vi "score.vi"() -> ()   [LabVIEW 2018]
panel:
  out "output array":bool[](array[boolean])
  out "Boolean 14":bool
  out "Boolean 13":bool
  out "Boolean 12":bool
  out "Boolean 11":bool
  out "Boolean 10":bool
  out "Boolean 9":bool
  out "Boolean 8":bool
  out "Boolean 7":bool
  out "Boolean 6":bool
  out "Boolean 5":bool
  out "Boolean 4":bool
  out "Boolean 3":bool
  out "Boolean 2":bool
  out "Boolean":bool
  out "Array":bool[][](array[boolean])=[[FALSE, FALSE, TRUE, FALSE, FALSE, FALSE, TRUE, FALSE, FALSE, FALSE], [TRUE, TRUE, FALSE, TRUE, FALSE, TRUE, TRUE, FALSE, FALSE, FALSE], [FALSE, TRUE, TRUE, TRUE, FALSE, TRUE, TRUE, FALSE, FALSE, FALSE], [FALSE, FALSE, TRUE, TRUE, TRUE, FALSE, TRUE, FALSE, FALSE, FALSE], [FALSE, TRUE, TRUE, TRUE, TRUE, TRUE, FALSE, FALSE, FALSE, FALSE], [TRUE, TRUE, TRUE, TRUE, TRUE, TRUE, FALSE, FALSE, FALSE, FALSE], [FALSE, FALSE, TRUE, FALSE, FALSE, TRUE, TRUE, TRUE, TRUE, TRUE], [TRUE, TRUE, TRUE, TRUE, TRUE, TRUE, TRUE, TRUE, TRUE, TRUE], [FALSE, TRUE, TRUE, TRUE, TRUE, TRUE, TRUE, TRUE, TRUE, TRUE]]
  in  "Numeric":dbl
  in  "stop":bool
  in  "time":dbl=60.0
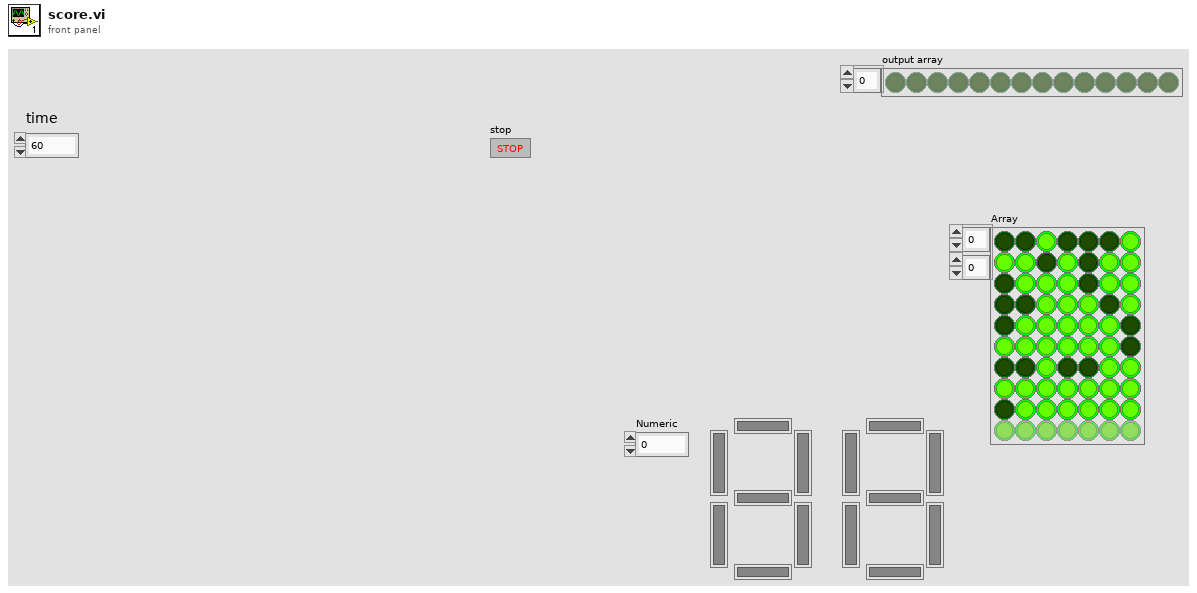
[diagram p1: front panel]
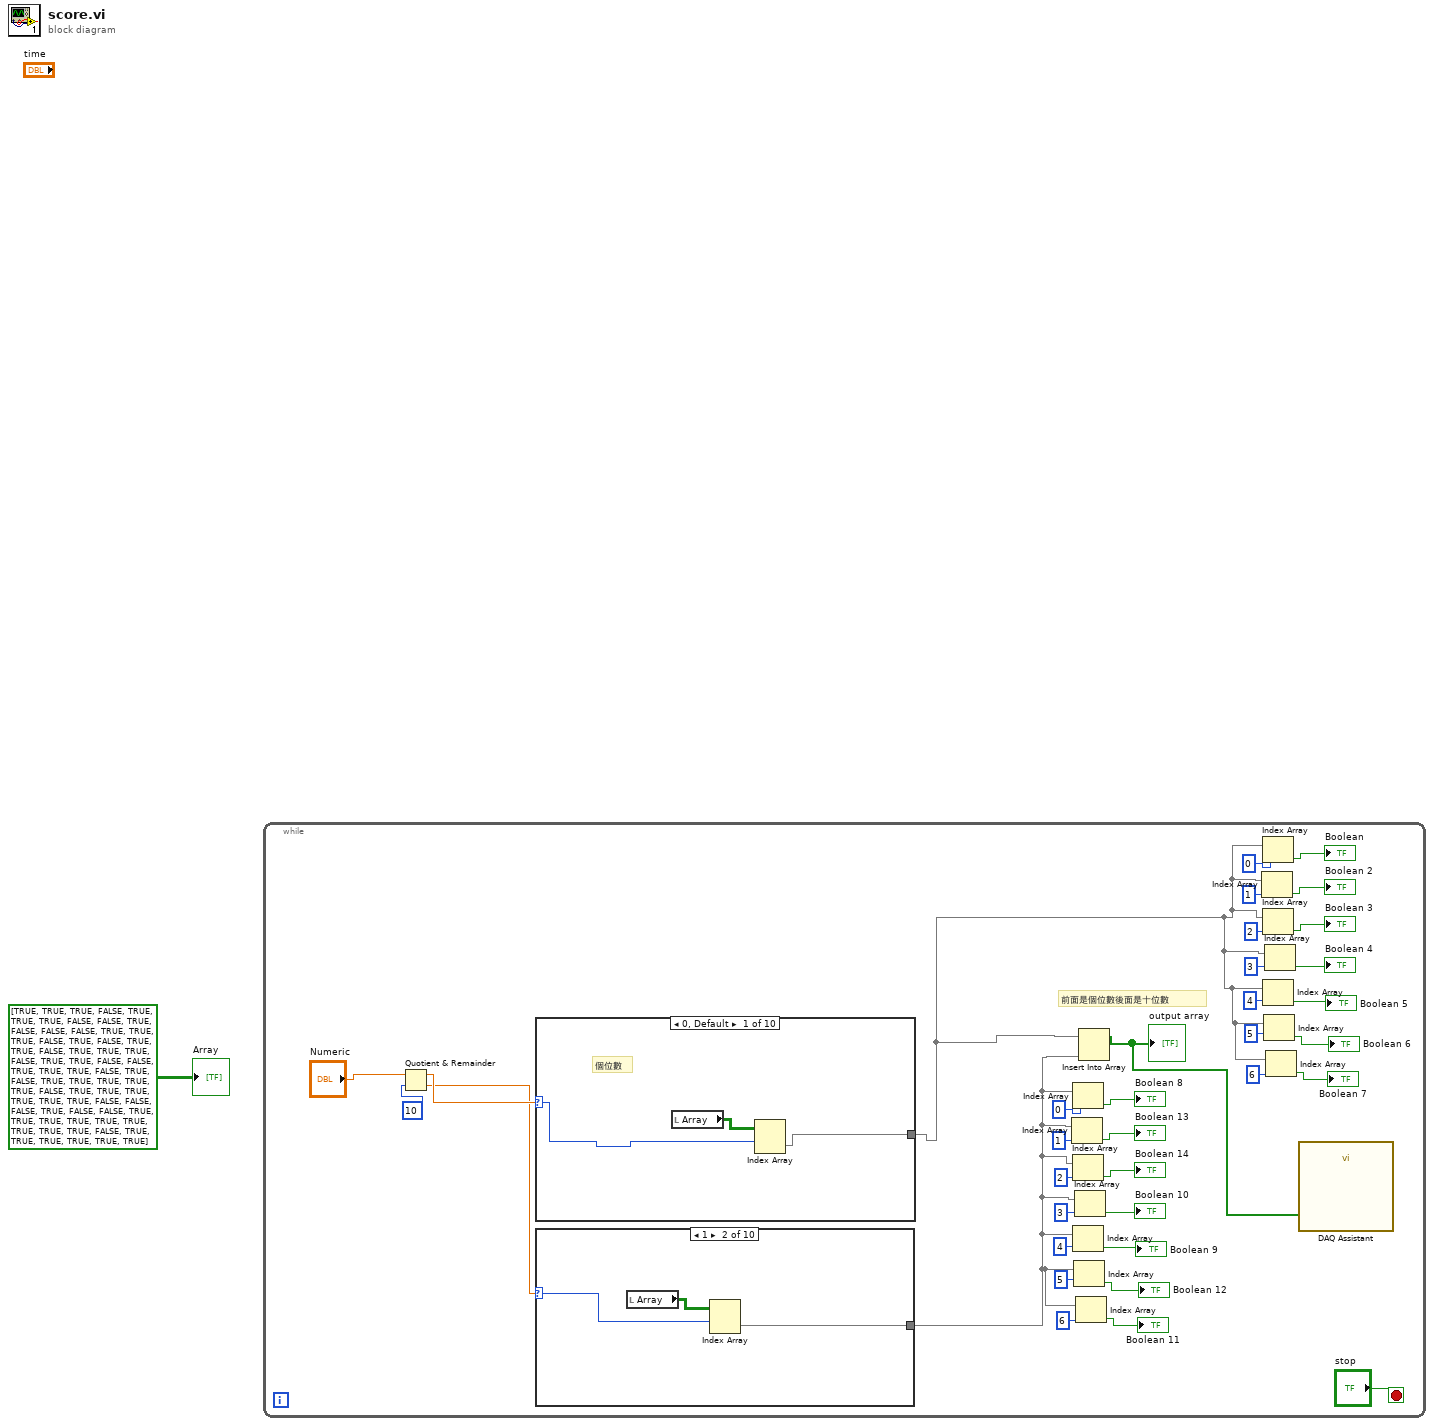
[diagram p0: block diagram]
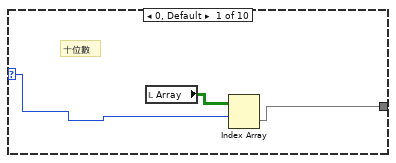
[diagram p2: hidden frame]
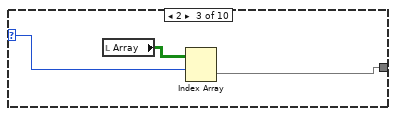
[diagram p3: hidden frame]
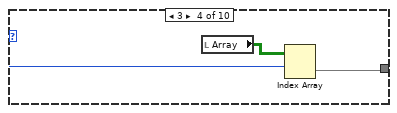
[diagram p4: hidden frame]
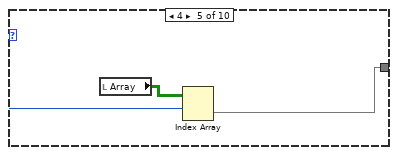
[diagram p5: hidden frame]
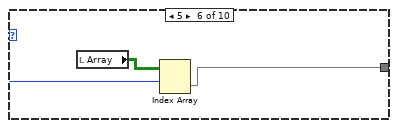
[diagram p6: hidden frame]
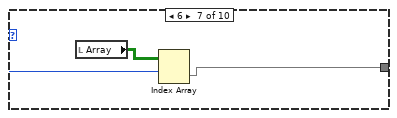
[diagram p7: hidden frame]
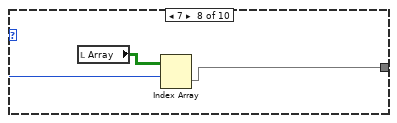
[diagram p8: hidden frame]
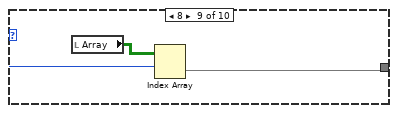
[diagram p9: hidden frame]
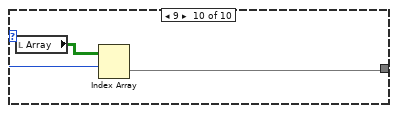
[diagram p10: hidden frame]
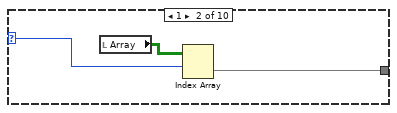
[diagram p11: hidden frame]
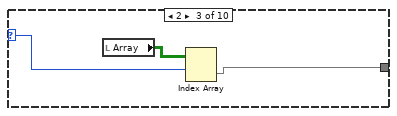
[diagram p12: hidden frame]
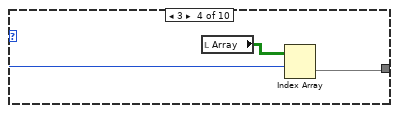
[diagram p13: hidden frame]
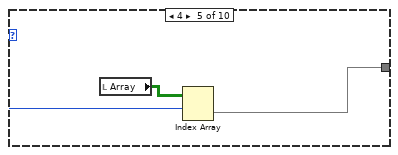
[diagram p14: hidden frame]
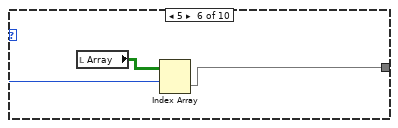
[diagram p15: hidden frame]
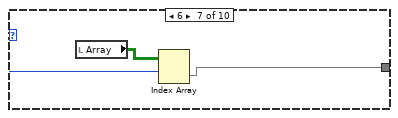
[diagram p16: hidden frame]
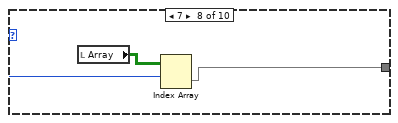
[diagram p17: hidden frame]
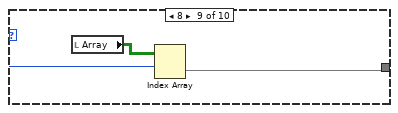
[diagram p18: hidden frame]
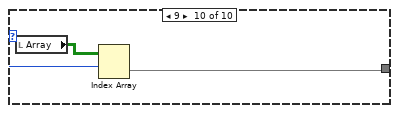
[diagram p19: hidden frame]
diagram:
  n1 = while {
    stop <- "stop" stop-if-true
    # "前面是個位數後面是十位數"
    n2 = Quotient & Remainder(x="Numeric", y=10) -> (x-y*floor(x/y)=w4:dbl, floor(x/y)=w3:dbl)
    n3 = case shown="0, Default" w4 {
      selector: w4 -> [w68 w72 w75 w78 w81 w84 w87 w90 w93 w96]
      tunnel: [w69 w71 w74 w77 w80 w83 w86 w89 w92 w95] -> w6
      frame 0, Default {
        # "個位數"
        n4 = local read "Array"() -> (w70:bool[][])
        n5 = Index Array(array=w70, index (row)=w68) -> (element=w69:bool[])  [unwired: 1 in]
      }
      frame 1 {
        n6 = local read "Array"() -> (w73:bool[][])
        n7 = Index Array(array=w73, index (row)=w72) -> (element=w71:bool[])  [unwired: 1 in]
      }
      frame 2 {
        n8 = local read "Array"() -> (w76:bool[][])
        n9 = Index Array(array=w76, index (row)=w75) -> (element=w74:bool[])  [unwired: 1 in]
      }
      frame 3 {
        n10 = local read "Array"() -> (w79:bool[][])
        n11 = Index Array(array=w79, index (row)=w78) -> (element=w77:bool[])  [unwired: 1 in]
      }
      frame 4 {
        n12 = local read "Array"() -> (w82:bool[][])
        n13 = Index Array(array=w82, index (row)=w81) -> (element=w80:bool[])  [unwired: 1 in]
      }
      frame 5 {
        n14 = local read "Array"() -> (w85:bool[][])
        n15 = Index Array(array=w85, index (row)=w84) -> (element=w83:bool[])  [unwired: 1 in]
      }
      frame 6 {
        n16 = local read "Array"() -> (w88:bool[][])
        n17 = Index Array(array=w88, index (row)=w87) -> (element=w86:bool[])  [unwired: 1 in]
      }
      frame 7 {
        n18 = local read "Array"() -> (w91:bool[][])
        n19 = Index Array(array=w91, index (row)=w90) -> (element=w89:bool[])  [unwired: 1 in]
      }
      frame 8 {
        n20 = local read "Array"() -> (w94:bool[][])
        n21 = Index Array(array=w94, index (row)=w93) -> (element=w92:bool[])  [unwired: 1 in]
      }
      frame 9 {
        n22 = local read "Array"() -> (w97:bool[][])
        n23 = Index Array(array=w97, index (row)=w96) -> (element=w95:bool[])  [unwired: 1 in]
      }
    }
    n24 = case shown="1" w3 {
      selector: w3 -> [w38 w42 w46 w49 w52 w55 w58 w61 w64 w67]
      tunnel: [w39 w41 w44 w47 w50 w53 w56 w59 w62 w65] -> w5
      frame 0, Default {
        # "十位數"
        n25 = local read "Array"() -> (w40:bool[][])
        n26 = Index Array(array=w40, index (row)=w38) -> (element=w39:bool[])  [unwired: 1 in]
      }
      frame 1 {
        n27 = local read "Array"() -> (w43:bool[][])
        n28 = Index Array(array=w43, index (row)=w42) -> (element=w41:bool[])  [unwired: 1 in]
      }
      frame 2 {
        n29 = local read "Array"() -> (w45:bool[][])
        n30 = Index Array(array=w45, index (row)=w46) -> (element=w44:bool[])  [unwired: 1 in]
      }
      frame 3 {
        n31 = local read "Array"() -> (w48:bool[][])
        n32 = Index Array(array=w48, index (row)=w49) -> (element=w47:bool[])  [unwired: 1 in]
      }
      frame 4 {
        n33 = local read "Array"() -> (w51:bool[][])
        n34 = Index Array(array=w51, index (row)=w52) -> (element=w50:bool[])  [unwired: 1 in]
      }
      frame 5 {
        n35 = local read "Array"() -> (w54:bool[][])
        n36 = Index Array(array=w54, index (row)=w55) -> (element=w53:bool[])  [unwired: 1 in]
      }
      frame 6 {
        n37 = local read "Array"() -> (w57:bool[][])
        n38 = Index Array(array=w57, index (row)=w58) -> (element=w56:bool[])  [unwired: 1 in]
      }
      frame 7 {
        n39 = local read "Array"() -> (w60:bool[][])
        n40 = Index Array(array=w60, index (row)=w61) -> (element=w59:bool[])  [unwired: 1 in]
      }
      frame 8 {
        n41 = local read "Array"() -> (w63:bool[][])
        n42 = Index Array(array=w63, index (row)=w64) -> (element=w62:bool[])  [unwired: 1 in]
      }
      frame 9 {
        n43 = local read "Array"() -> (w66:bool[][])
        n44 = Index Array(array=w66, index (row)=w67) -> (element=w65:bool[])  [unwired: 1 in]
      }
    }
    n45 = Index Array(array=w5, index=1) -> (element=→"Boolean 13":bool)
    n46 = Index Array(array=w5, index=0) -> (element=→"Boolean 8":bool)
    n47 = Index Array(array=w5, index=2) -> (element=→"Boolean 14":bool)
    n48 = Index Array(array=w5, index=4) -> (element=→"Boolean 9":bool)
    n49 = Index Array(array=w5, index=5) -> (element=→"Boolean 12":bool)
    n50 = Index Array(array=w5, index=3) -> (element=→"Boolean 10":bool)
    n51 = Index Array(array=w5, index=6) -> (element=→"Boolean 11":bool)
    n52 = Insert Into Array(array=w6, new element=w5) -> (w2:bool[])  [unwired: 1 in]
    "output array" <- w2
    n53 = Index Array(array=w6, index=1) -> (element=→"Boolean 2":bool)
    n54 = Index Array(array=w6, index=0) -> (element=→"Boolean":bool)
    n55 = Index Array(array=w6, index=2) -> (element=→"Boolean 3":bool)
    n56 = Index Array(array=w6, index=4) -> (element=→"Boolean 5":bool)
    n57 = Index Array(array=w6, index=5) -> (element=→"Boolean 6":bool)
    n58 = Index Array(array=w6, index=3) -> (element=→"Boolean 4":bool)
    n59 = Index Array(array=w6, index=6) -> (element=→"Boolean 7":bool)
    n60 = call "DAQ Assistant"("data"=w2) -> ()  [unwired: 17 in, 2 out]
  }
  "Array" <- bool[][] [[TRUE, TRUE, TRUE, FALSE, TRUE, TRUE, TRUE], [FALSE, FALSE, TRUE, FALSE, FALSE, FALSE, TRUE], [TRUE, TRUE, FALSE, TRUE, FALSE, TRUE, TRUE], [FALSE, TRUE, TRUE, TRUE, FALSE, TRUE, TRUE], [FALSE, FALSE, TRUE, TRUE, TRUE, FALSE, TRUE], [FALSE, TRUE, TRUE, TRUE, TRUE, TRUE, FALSE], [TRUE, TRUE, TRUE, TRUE, TRUE, TRUE, FALSE], [FALSE, FALSE, TRUE, FALSE, FALSE, TRUE, TRUE], [TRUE, TRUE, TRUE, TRUE, TRUE, TRUE, TRUE], [FALSE, TRUE, TRUE, TRUE, TRUE, TRUE, TRUE]]
